vi "ArrayGlobal.vi"(0 "Function":T1(ring), 1 "ArrrayIn":u16[][](array[numeric]), 3 "Start index Y":u32, 4 "Start index X":u32, 5 "Slide":u32) -> (15 "ArrayOut":u16[][](array[numeric]), 18 "SubarrayOut":u16[](array[numeric]))   [LabVIEW 2017]
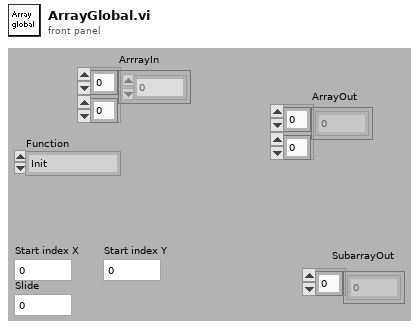
[diagram p1: front panel]
types:
  T1 = enum16{"Init", "Write", "Read array", "Read subarray"}
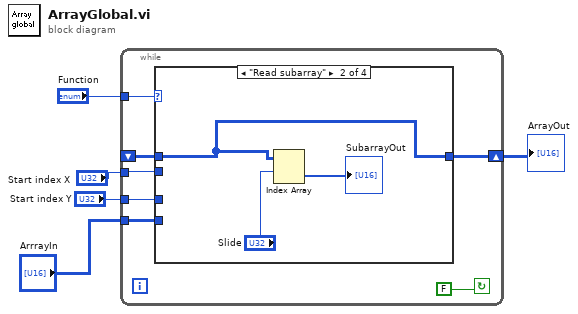
[diagram p0: block diagram]
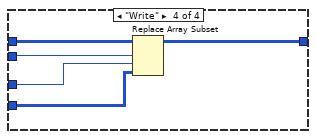
[diagram p4: hidden frame]
diagram:
  n1 = while {
    tunnel: "Function" -> [w12]
    shift-right: [w11] -> w2
    shift-left: _ -> [w10]
    tunnel: "Start index X" -> [w9]
    tunnel: "ArrrayIn" -> [w8]
    tunnel: "Start index Y" -> [w6]
    stop <- FALSE continue-if-true
    n2 = case shown="\"Read subarray\"" w12 {
      tunnel: [w13 w15 w17 w20] -> w11
      tunnel: w10 -> [_ w15 w17 w22]
      tunnel: w9 -> [_ _ _ w19]
      tunnel: w8 -> [w13 _ _ w21]
      tunnel: w6 -> [_ _ _ w18]
      frame "Init", Default {
        # "make here an reshape array like in the printouts"
      }
      frame "Read subarray" {
        n3 = Index Array(array=w15, index (row)="Slide") -> (element=→"SubarrayOut":u16[])  [unwired: 1 in]
      }
      frame "Read array" {
      }
      frame "Write" {
        n4 = Replace Array Subset(array=w22, new element=w21, index (row)=w19, index (col)=w18) -> (w20:u16[][])
      }
    }
  }
  "ArrayOut" <- w2
